vi "Add a Blank View.vi"(8 "error in (no error)":errorcluster, 10 "TabCtls":refnum<vi>[](array[refnum]), 11 "Coords":T1) -> (0 "error out":errorcluster)   [LabVIEW 2020, in "MDI ViewManager.lvlib"]
uses:
  MDI ViewManager.lvlib
  <vilib>/Utility/miscctls.llb/LVPoint32TypeDef.ctl
  <vilib>/Utility/miscctls.llb/LVBoundsTypeDef.ctl
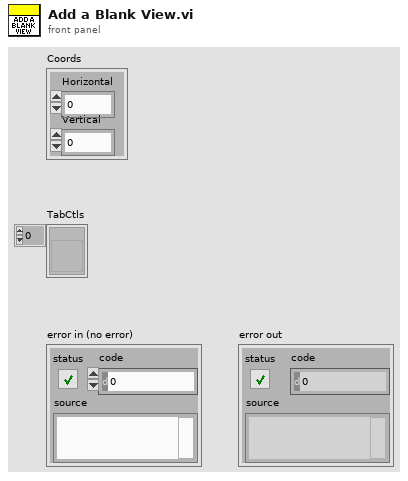
[diagram p1: front panel]
types:
  T1 = typedef "LVPoint32TypeDef.ctl" = cluster{"Horizontal":i32, "Vertical":i32}
  T2 = typedef "LVBoundsTypeDef.ctl" = cluster{"Width":u32, "Height":u32}
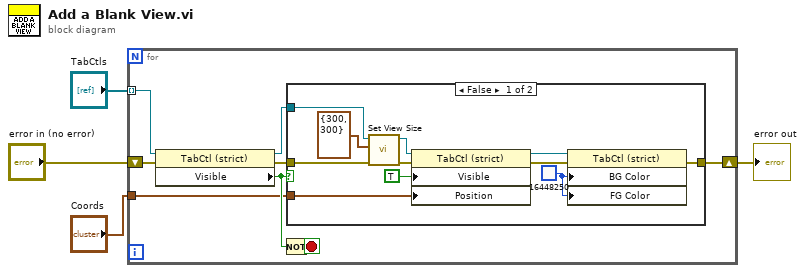
[diagram p0: block diagram]
diagram:
  n1 = for {
    tunnel: "TabCtls" -> [w12] mode=indexing
    tunnel: "Coords" -> [w8]
    shift-right: [w5] -> w1
    shift-left: "error in (no error)" -> [w6]
    stop <- w10 stop-if-true
    n2 = property class="TabCtl (strict)"(reference=w12, error in=w6) -> (reference out=w9:refnum<vi>, error out=w7:errorcluster, "Visible"=w11:bool)
    n3 = Not(x=w11) -> (.not. x?=w10:bool)
    n4 = case shown="False" w11 {
      tunnel: w9 -> [w21 _]
      tunnel: w8 -> [w22 _]
      tunnel: w7 -> [w14 w24]
      tunnel: [w13 w24] -> w5
      frame False {
        w17 = u32 16448250 ("Colors:BG Color")
        n5 = call "Set View Size.vi"("error in (no error)"=w14, "TabDimension"=T2 {"Width"=300, "Height"=300}, "TabControlRef in"=w21) -> ("error out"=w15:errorcluster, "TabControlRef out"=w20:refnum<vi>)  [unwired: 7 in]
        n6 = property class="TabCtl (strict)"(reference=w20, error in=w15, "Visible"=TRUE, "Position"=w22) -> (reference out=w18:refnum<vi>, error out=w16:errorcluster)
        n7 = property class="TabCtl (strict)"(reference=w18, error in=w16, "BG Color"=w17, "FG Color"=w17) -> (error out=w13:errorcluster)  [unwired: 1 out]
      }
      frame True {
      }
    }
  }
  "error out" <- w1
